vi "UE9 Efunction Loop Example.vi"() -> (0 "error out":errorcluster)   [LabVIEW 2021]
panel:
  in  "FirstFound":bool=TRUE
  in  "ConnectionType":u16(ring) items=["LJ_ctUSB", "LJ_ctETHERNET"]
  in  "Address":string="192.168.1.209"
  out "AIN1 Voltage":dbl format="%.6f"
  in  "stop":bool
  in  "Interval (ms)":u32=500
  out "FIO1 State In":bool
  in  "DAC0 Voltage":dbl format="%.3f"
  in  "FIO2 State Out":bool
  out "Error Message":string
  out "AIN0 Voltage":dbl format="%.6f"
  # "Sets DAC0, sets FIO2, reads AIN0, reads AIN1, and reads FIO1."
  # "Specify an IP address for Ethernet, or Local ID\nfor USB.  If FirstFound is selected, Local ID is\nignored for USB."
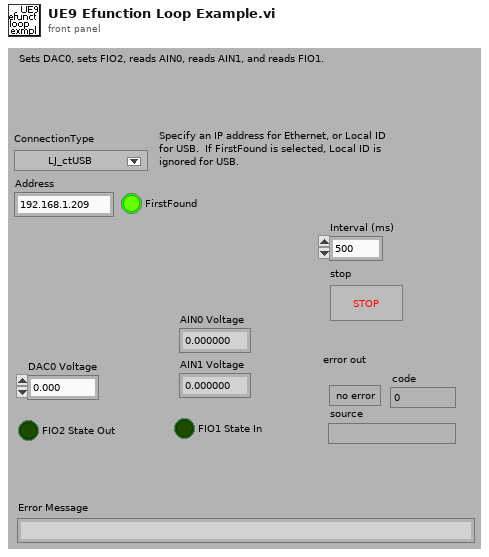
[diagram p1: front panel]
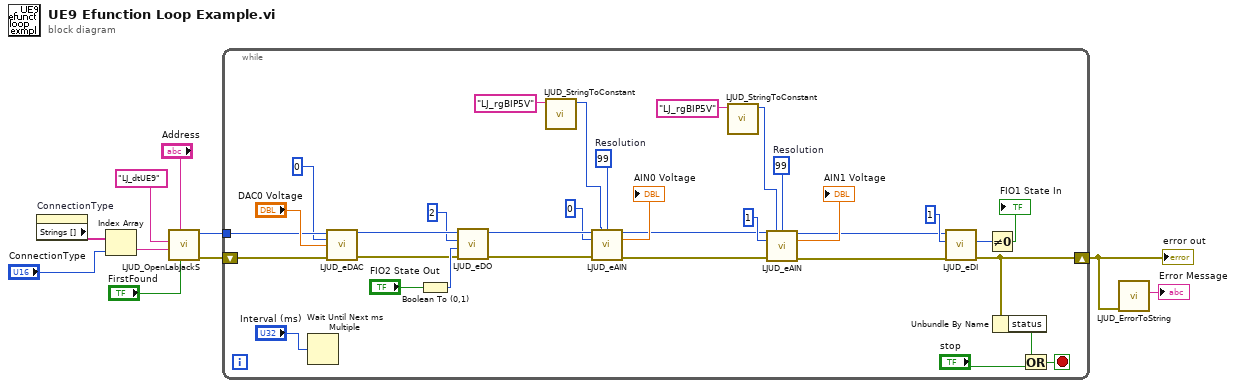
[diagram p0: block diagram]
diagram:
  n1 = property on="ConnectionType" class="Ring (strict)"() -> ("Strings []"=w3:string[])  [unwired: 2 in, 2 out]
  n2 = Index Array(array=w3, index="ConnectionType") -> (element=w2:string)
  n3 = call "LJUD_OpenLabJackS.vi"("FirstFound"="FirstFound", "Address"="Address", "ConnectionType"=w2, "DeviceType"="LJ_dtUE9") -> ("error out"=w6:errorcluster, "Handle"=w8:i32)  [unwired: 5 in, 1 out]
  n4 = while {
    shift-left: w6 -> [w24]
    shift-right: [w25] -> w7
    tunnel: w8 -> [w38]
    stop <- w27 stop-if-true
    w17 = 99  # Resolution
    w18 = 99  # Resolution
    n5 = Wait Until Next ms Multiple(millisecond multiple="Interval (ms)") -> ()  [unwired: 1 out]
    n6 = call "LJUD_eDAC.vi"("Handle In"=w38, "Channel"=0, "Voltage"="DAC0 Voltage", "error in"=w24) -> ("Handle Out"=w36:i32, "error out"=w37:errorcluster)  [unwired: 10 in]
    n7 = Boolean To (0,1)(Boolean="FIO2 State Out") -> (0, 1=w41:i16)
    n8 = call "LJUD_eDO.vi"("error in"=w37, "State"=w41, "Channel"=2, "Handle In"=w36) -> ("error out"=w35:errorcluster, "Handle Out"=w34:i32)  [unwired: 6 in]
    n9 = call "LJUD_StringToConstant.vi"("String"="LJ_rgBIP5V") -> ("Constant Number"=w13:i32)  [unwired: 9 in, 1 out]
    n10 = call "LJUD_eAIN.vi"("Handle In"=w34, "Range"=w13, "Resolution"=w18, "ChannelP"=0, "error in"=w35) -> ("Handle Out"=w16:i32, "Voltage"=→"AIN0 Voltage":dbl, "error out"=w21:errorcluster)  [unwired: 8 in]
    n11 = call "LJUD_StringToConstant.vi"("String"="LJ_rgBIP5V") -> ("Constant Number"=w11:i32)  [unwired: 9 in, 1 out]
    n12 = call "LJUD_eAIN.vi"("Handle In"=w16, "Range"=w11, "Resolution"=w17, "ChannelP"=1, "error in"=w21) -> ("Handle Out"=w15:i32, "Voltage"=→"AIN1 Voltage":dbl, "error out"=w20:errorcluster)  [unwired: 8 in]
    n13 = call "LJUD_eDI.vi"("error in"=w20, "Channel"=1, "Handle In"=w15) -> ("error out"=w25:errorcluster, "State"=w42:i32)  [unwired: 6 in, 1 out]
    n14 = Not Equal To 0?(x=w42) -> (x != 0?=→"FIO1 State In":bool)
    n15 = Unbundle By Name(w25) -> ("status"=w26:bool)
    n16 = Or(x=w26, y="stop") -> (x .or. y?=w27:bool)
  }
  "error out" <- w7
  n17 = call "LJUD_ErrorToString.vi"("error in"=w7) -> ("String"=→"Error Message":string)  [unwired: 10 in]
